vi "Get Server State Ref.vi"(11 "gRPC server in":refnum<class "Servicer.lvclass">) -> (2 "Server State Ref":refnum<data-value>, 3 "gRPC server out":refnum<class "Servicer.lvclass">)   [LabVIEW 2019, in "gRPC-servicer.lvlib" / "Servicer.lvclass"]
uses:
  Servicer.lvclass
  typeDefs/Server State Data.ctl
  Servicer.lvclass/Servicer.ctl
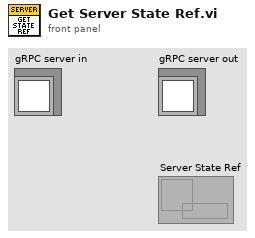
[diagram p1: front panel]
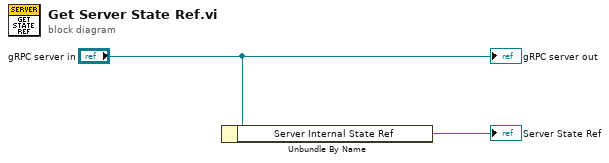
[diagram p0: block diagram]
diagram:
  n1 = Unbundle By Name("gRPC server in") -> ("Server Internal State Ref"=→"Server State Ref":refnum<data-value>)
  "gRPC server out" <- "gRPC server in"
